vi "FT_Set_DTR.vi"(0 "Handle":u32) -> (1 "Handle 2":u32, 2 "FT_Status":u32)   [LabVIEW 2011]
uses:
  FTD2XX.dll
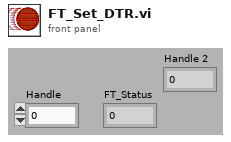
[diagram p1: front panel]
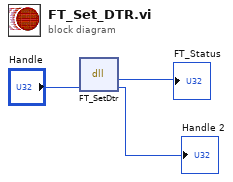
[diagram p0: block diagram]
diagram:
  n1 = dll-call lib="D:/WORK/LabView/#Avesta/D2XX_Functions_7.0/FTD2XX.dll" fn="FT_SetDtr" label="FT_SetDTR"("Handle"="Handle") -> ("FT_Status"=→"FT_Status":u32, "Handle"=→"Handle 2":u32)  [unwired: 3 in, 2 out]
